vi "ScanParam2DAQParam_old.vi"(11 "AOL_Globals":T1={"Imaging Protocol"=enum."AOL Z-Stack", "Number of POI"=0, "Number of Miniscans"=0, "Number of Trials"=0, "Number of Cycles "=0, "# Averaged Frames"=0, "Laser power (%)"=0, "Pockels (V)"=0.0, "Acquisition Length (sec)"=0.0, "Fill time (us)"=0.0, "POI Dwell time (us)"=0.0, "Miniscan Dwell time per pixel (us)"=0.0, "PMT 1"=0.0, "PMT 2"=0.0, "Back Apperture (mA)"=200.0, "Frame Size"=0, "Center Frequency"=0.0, "Field of View (norm)"=0.0, "DwellTime (us)"=0.0, "Wavelength (nm)"=0.0, "Zoom"=0.0, "AOL Z"=0.0, "AOL Mode"=enum."Raster", "GridXY"=0.0, "GridZ"=0.0, "TriggerPeriod (sec)"=0.0, "Number of Pixels in Miniscan"=0, "Experiment folder path"=path "", "X centre"=0.0, "Y centre"=0.0, "Angle (degrees)"=0.0, "Plane Mode"=0, "Threshold"=[], "Regenerate Chirps"=FALSE, "Rectangle ROI length (pixels)"=0, "Rectangle ROI height (pixels)"=0, "AOD fill"=4900, "StartupDelay"=0, "Samples Wait after Trigger"=5080, "Slip Cycle"=600000, "Add Cycle"=TRUE, "Functional Mode"=enum."Point", "Z Start"=0.0, "Z Stop"=0.0, "# Planes"=0, "Total Pixels"=0, "Variable Miniscan Pixels"=[], "Use Variable Length"=FALSE, "Use Variable Resolution"=FALSE, "Laser power (%) at Z Start"=0, "Laser power (%) at Z Stop"=0, "Ref Z Step"=0, "Ref Dwell Time (us)"=0.0, "Field of View (um)"=175.0} {"Plane Mode" items=["XY Plane", "XZ Plane", "YZ Plane", "arbitraryplane"]; "Frame Size" items=["100X100"=100, "128X128"=128, "200X200"=200, "256X256"=256, "512X512"=512, "1024x1024"=1024, "2048x2048"=2048]; "Back Apperture (mA)" format="%#.6g"; "Pockels (V)" format="%#.6g"; "PMT 2" format="%#.6g"; "PMT 1" format="%#.6g"; "Angle (degrees)" format="%#.6g"; "POI Dwell time (us)" format="%#.6g"}) -> (3 "DAQ Input Parameters(FlexRIO)":T7 {"diff_threshZ" format="%#_11g"; "proportioanl_scale Z" format="%#_15g"; "var_x" format="%#_14g"; "var_y" format="%#_14g"; "scale" format="%#_15g"; "diff_thresh" format="%#_11g"; "proportioanl_scale" format="%#_15g"})   [LabVIEW 2020]
uses:
  AOLdrivers/Controls/UI Imaging Parameters.ctl
  Typedefs/Controls/DAQ Input Parameters(FlexRIO).ctl
  FPGA DAQ/FPGA Typedefs/scan_typr.ctl
  Movement Correction/Typedefs/Control algorithm.ctl
  Typedefs/Controls/AOL_Globals.ctl
  Typedefs/Imaging Protocols enum.ctl
  Typedefs/Frame Size.ctl
  Typedefs/AOL modes.ctl
  Typedefs/Plane Mode.ctl
  Typedefs/Functional Mode.ctl
panel:
  in  "Samples Wait after Trigger(240 MHz)":u16=5500
  in  "AOD fill(240 MHz)":u16=4900
  in  "UI Imaging Parameters":T10={"Frame Size"=200, "Dwell Time (ms)"=0.0, "Wavelength (nm)"=0.0, "Zoom"=0.0, "AOL Mode"=enum."Raster Scanning", "Field of View"=4.35, "Imaging Mode"=enum."Live Imaging", "AOL Z"=0.0, "Averages"=0.0} {"Field of View" items=["FOV1"=4.35, "FOV 2"=5.8, "FOV 3"=8.7]; "Frame Size" items=["20X20"=0, "100X100"=100, "128X128"=128, "200X200"=200, "256X256"=256, "512X512"=512]}
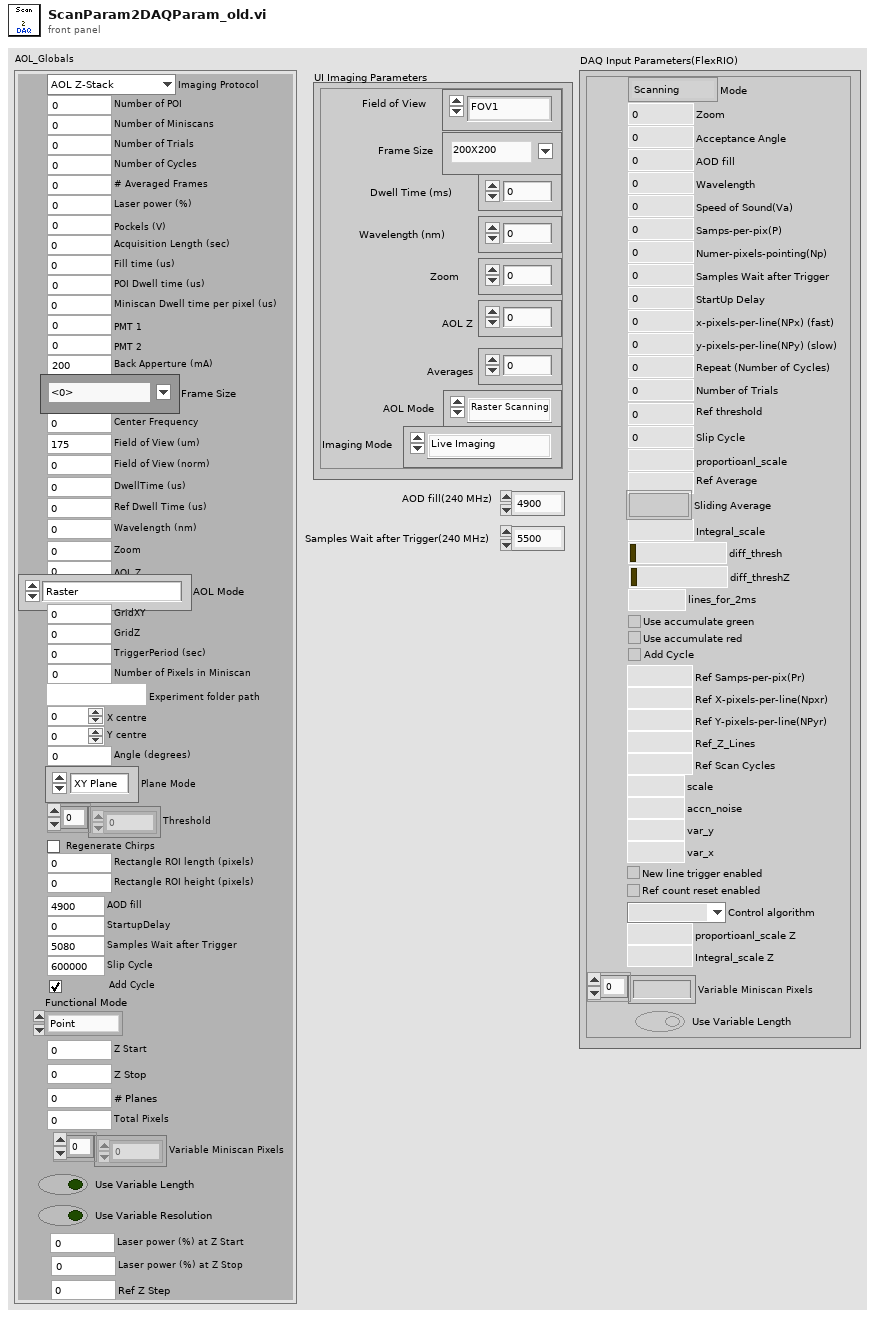
[diagram p1: front panel]
types:
  T1 = typedef "AOL_Globals.ctl" = cluster{"Imaging Protocol":T2, "Number of POI":u16, "Number of Miniscans":u16, "Number of Trials":u16, "Number of Cycles ":u64, "# Averaged Frames":u16, "Laser power (%)":u8, "Pockels (V)":dbl, "Acquisition Length (sec)":dbl, "Fill time (us)":dbl, "POI Dwell time (us)":dbl, "Miniscan Dwell time per pixel (us)":dbl, "PMT 1":dbl, "PMT 2":dbl, "Back Apperture (mA)":dbl, "Frame Size":T3, "Center Frequency":dbl, "Field of View (norm)":dbl, "DwellTime (us)":dbl, "Wavelength (nm)":dbl, "Zoom":dbl, "AOL Z":dbl, "AOL Mode":T4, "GridXY":dbl, "GridZ":dbl, "TriggerPeriod (sec)":dbl, "Number of Pixels in Miniscan":u16, "Experiment folder path":path, "X centre":dbl, "Y centre":dbl, "Angle (degrees)":dbl, "Plane Mode":T5, "Threshold":u16[], "Regenerate Chirps":bool, "Rectangle ROI length (pixels)":u16, "Rectangle ROI height (pixels)":u16, "AOD fill":u16, "StartupDelay":i32, "Samples Wait after Trigger":u16, "Slip Cycle":u32, "Add Cycle":bool, "Functional Mode":T6, "Z Start":dbl, "Z Stop":dbl, "# Planes":i32, "Total Pixels":i32, "Variable Miniscan Pixels":u16[], "Use Variable Length":bool, "Use Variable Resolution":bool, "Laser power (%) at Z Start":u8, "Laser power (%) at Z Stop":u8, "Ref Z Step":i8, "Ref Dwell Time (us)":dbl, "Field of View (um)":dbl}
  T2 = typedef "Imaging Protocols enum.ctl" = enum16{"AOL Z-Stack", "Motor Z Stack", "Functional Acquisition", "Single Plane Acquisition", "Volume Acquisition", "Live Imaging", "Live Plane Imaging", "Live Volume Imaging"}
  T3 = typedef "Frame Size.ctl" = u16
  T4 = typedef "AOL modes.ctl" = enum16{"Raster", "Structural", "Pointing", "Mini Scan", "Alignment"}
  T5 = typedef "Plane Mode.ctl" = u16
  T6 = typedef "Functional Mode.ctl" = enum16{"Point", "Line", "Patch", "Plane", "Volume"}
  T7 = typedef "DAQ Input Parameters(FlexRIO).ctl" = cluster{"Mode":T8, "Zoom":i8, "Acceptance Angle":i8, "AOD fill":u16, "Wavelength":i16, "Speed of Sound(Va)":i8, "Samps-per-pix(P)":i16, "Numer-pixels-pointing(Np)":u32, "Samples Wait after Trigger":u16, "StartUp Delay":i32, "x-pixels-per-line(NPx) (fast)":u16, "y-pixels-per-line(NPy) (slow)":u16, "Repeat (Number of Cycles)":u32, "Number of Trials":u16, "Ref threshold":u16, "Slip Cycle":u32, "proportioanl_scale":fxp<+,16,2>, "Ref Average":u16, "Sliding Average":bool, "Integral_scale":fxp<+/-,16,12>, "diff_thresh":fxp<+/-,16,8>, "diff_threshZ":fxp<+/-,16,8>, "lines_for_2ms":i16, "Use accumulate green":bool, "Use accumulate red":bool, "Add Cycle":bool, "Ref Samps-per-pix(Pr)":i16, "Ref X-pixels-per-line(Npxr)":i16, "Ref Y-pixels-per-line(NPyr)":i16, "Ref_Z_Lines":i16, "Ref Scan Cycles":i32, "scale":fxp<+,16,2>, "accn_noise":fxp<+,16,16>, "var_y":fxp<+,16,4>, "var_x":fxp<+,16,4>, "New line trigger enabled":bool, "Ref count reset enabled":bool, "Control algorithm":T9, "proportioanl_scale Z":fxp<+,16,2>, "Integral_scale Z":fxp<+/-,16,12>, "Variable Miniscan Pixels":u16[], "Use Variable Length":bool}
  T8 = typedef "scan_typr.ctl" = enum16{"Scanning", "Pointing", "Pointing & MC", "Scanning & MC"}
  T9 = typedef "Control algorithm.ctl" = enum16{"PID", "Kalman"}
  T10 = typedef "UI Imaging Parameters.ctl" = cluster{"Frame Size":u16, "Dwell Time (ms)":dbl, "Wavelength (nm)":dbl, "Zoom":dbl, "AOL Mode":enum16{"Raster Scanning", "Structural Imaging", "Functional Imaging", "Alignment Mode", "Mini Scan"}, "Field of View":sgl, "Imaging Mode":enum16{"Live Imaging", "AOL Zstack", "Motor Zstack", "Functional Imaging"}, "AOL Z":sgl, "Averages":dbl}
  T11 = enum16{"Raster Scanning", "Structural Imaging", "Functional Imaging", "Alignment Mode", "Mini Scan"}
  T12 = enum16{"Scanning", "Pointing", "Pointing & MC", "Scanning & MC"}
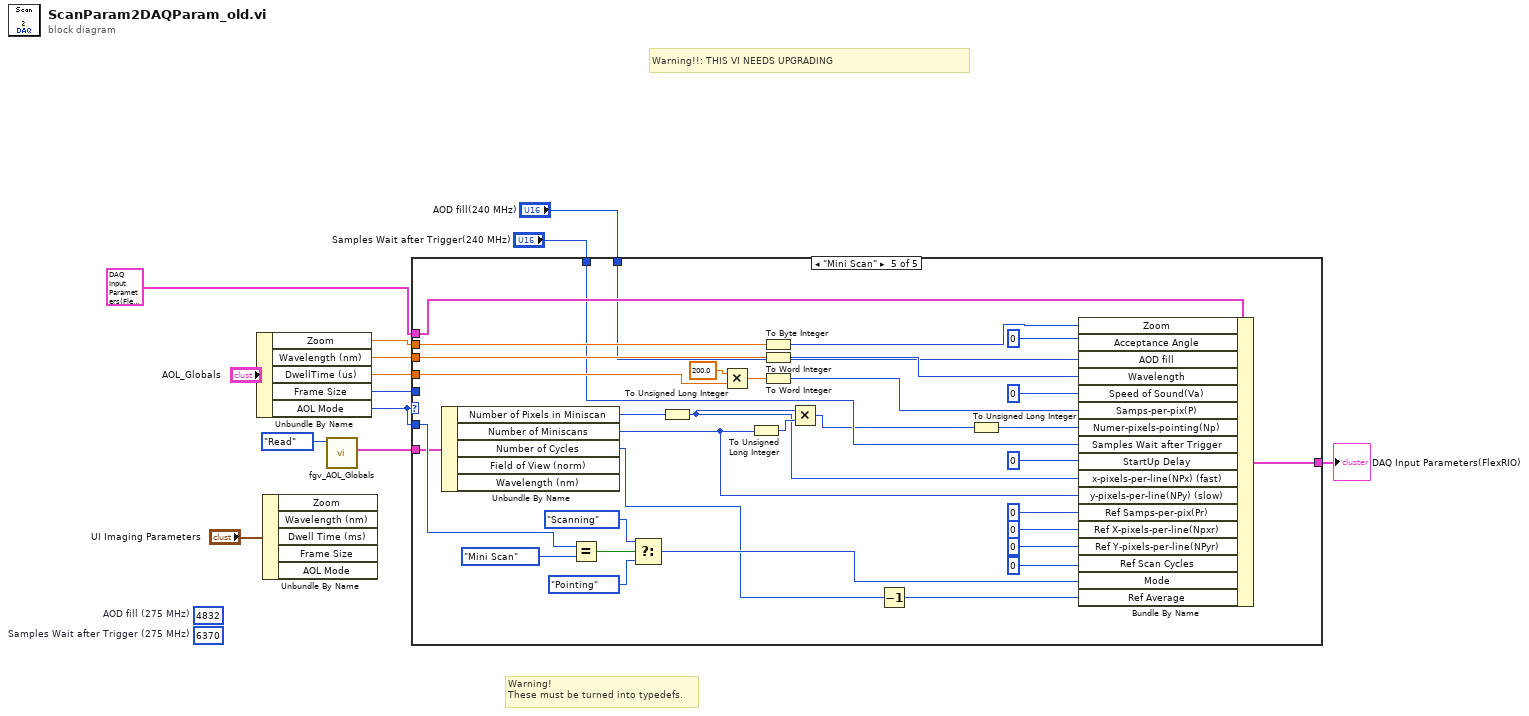
[diagram p0: block diagram]
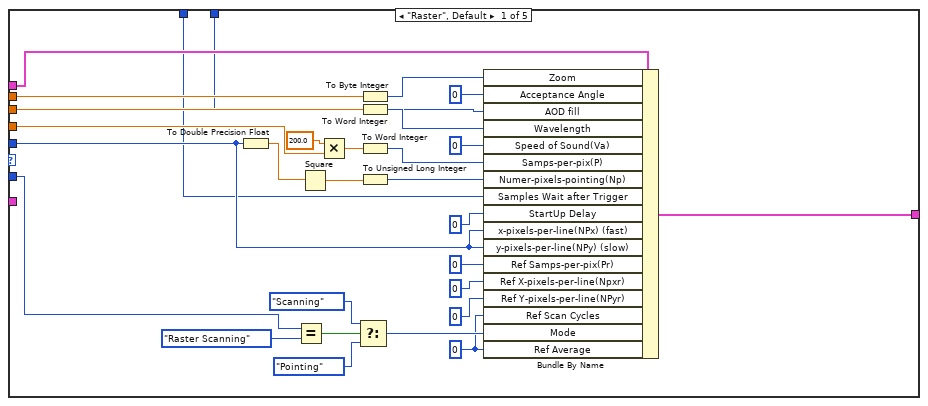
[diagram p2: hidden frame]
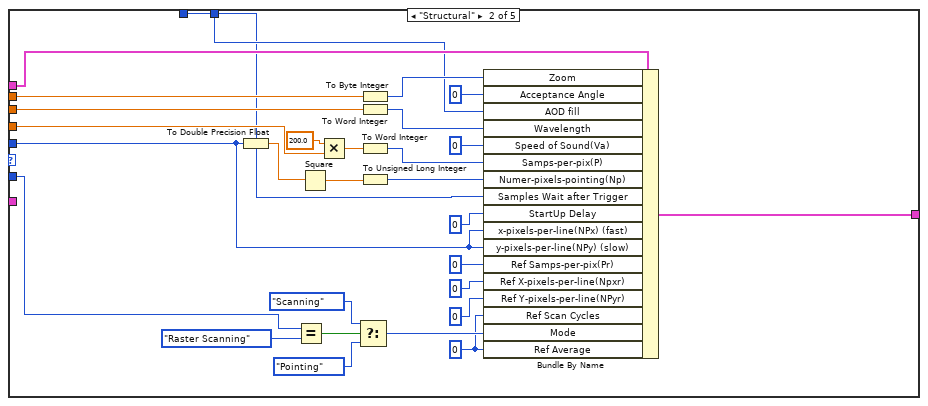
[diagram p3: hidden frame]
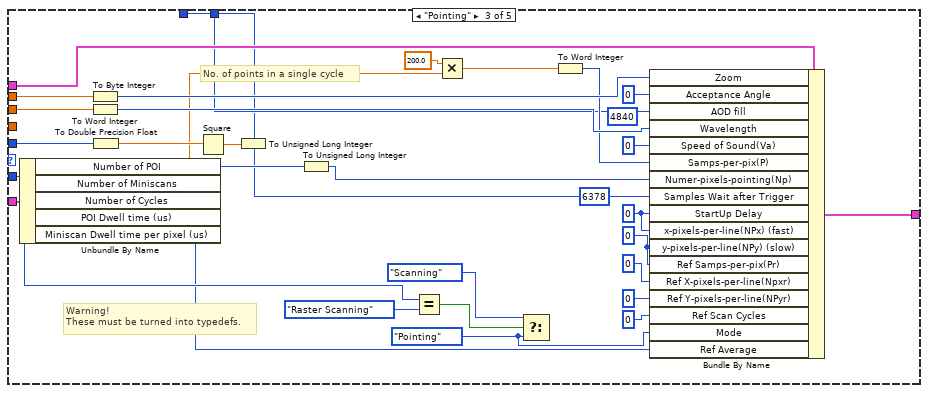
[diagram p4: hidden frame]
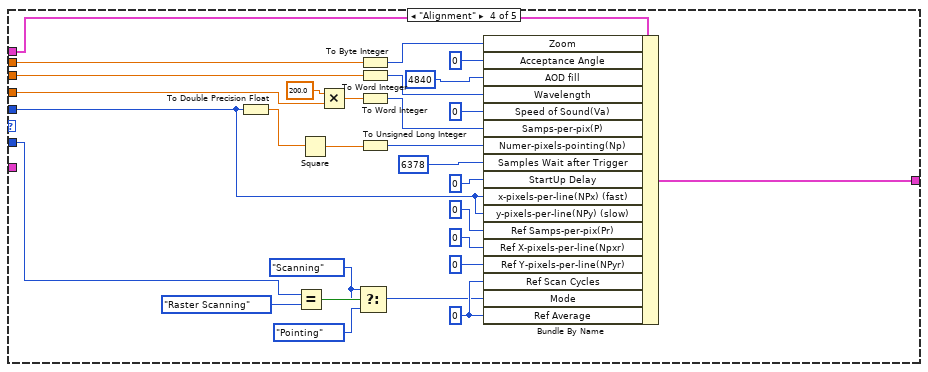
[diagram p5: hidden frame]
diagram:
  (unwired) u16 6370  # Samples Wait after Trigger (275 MHz)
  (unwired) u16 4832  # AOD fill (275 MHz)
  # "Warning!!: THIS VI NEEDS UPGRADING"
  # "Warning!\nThese must be turned into typedefs."
  n1 = Unbundle By Name("AOL_Globals") -> ("Zoom"=w8:dbl, "Wavelength (nm)"=w7:dbl, "DwellTime (us)"=w6:dbl, "Frame Size"=w5:T3, "AOL Mode"=w4:T4)
  n2 = Unbundle By Name("UI Imaging Parameters") -> ()  [unwired: 5 out]
  n3 = call "fgv_AOL_Globals.vi"("Function"=enum16{"Intialize", "Write", "Read", "Clear"}."Read") -> ("AOL_Globals"=w3:T1)  [unwired: 9 in, 1 out]
  n4 = case shown="\"Mini Scan\"" w4 {
    tunnel: T7 data[162B] ("DAQ Input Parameters(FlexRIO)") -> [w42 w71 w102 w106 w164]
    tunnel: w4 -> [w31 w60 w94 w121 w154]
    tunnel: [w29 w58 w92 w119 w152] -> w11
    tunnel: w8 -> [w22 w51 w86 w112 w149]
    tunnel: w6 -> [w20 w49 _ w110 w148]
    tunnel: w7 -> [w19 w48 w84 w109 w147]
    tunnel: w5 -> [w18 w47 w83 w108 _]
    tunnel: w3 -> [_ _ w80 _ w144]
    tunnel: "AOD fill(240 MHz)" -> [w15 w44 w73 _ w141]
    tunnel: "Samples Wait after Trigger(240 MHz)" -> [w14 w43 w72 _ w140]
    frame "Raster", Default {
      w16 = 0 ("Ref Scan Cycles")
      n5 = To Double Precision Float(number=w18) -> (double precision float=w24:dbl)
      n6 = Equal?(x=w31, y=T11."Raster Scanning" ("AOL Mode")) -> (x = y?=w30:bool)
      n7 = Square(x=w24) -> (x^2=w28:dbl)
      n8 = Multiply(x=200.0, y=w20) -> (x*y=w27:dbl)
      n9 = Select(t=T12."Scanning" ("Mode"), s=w30, f=T12."Pointing" ("Mode")) -> (s? t:f=w17:T12)
      n10 = To Byte Integer(number=w22) -> (8bit integer=w41:i8)
      n11 = To Word Integer(number=w19) -> (16bit integer=w40:i16)
      n12 = To Word Integer(number=w27) -> (16bit integer=w25:i16)
      n13 = To Unsigned Long Integer(number=w28) -> (unsigned 32bit integer=w23:u32)
      n14 = Bundle By Name(cluster=w42, "Zoom"=w41, "Acceptance Angle"=i8 0, "AOD fill"=w15, "Wavelength"=w40, "Speed of Sound(Va)"=i8 0, "Samps-per-pix(P)"=w25, "Numer-pixels-pointing(Np)"=w23, "Samples Wait after Trigger"=w14, "StartUp Delay"=0, "x-pixels-per-line(NPx) (fast)"=w18, "y-pixels-per-line(NPy) (slow)"=w18, "Ref Samps-per-pix(Pr)"=i16 0, "Ref X-pixels-per-line(Npxr)"=i16 0, "Ref Y-pixels-per-line(NPyr)"=i16 0, "Ref Scan Cycles"=w16, "Mode"=w17, "Ref Average"=w16) -> (w29:T7)
    }
    frame "Structural" {
      w45 = 0 ("Ref Scan Cycles")
      n15 = To Double Precision Float(number=w47) -> (double precision float=w53:dbl)
      n16 = Equal?(x=w60, y=T11."Raster Scanning" ("AOL Mode")) -> (x = y?=w59:bool)
      n17 = Square(x=w53) -> (x^2=w57:dbl)
      n18 = Multiply(x=200.0, y=w49) -> (x*y=w56:dbl)
      n19 = Select(t=T12."Scanning" ("Mode"), s=w59, f=T12."Pointing" ("Mode")) -> (s? t:f=w46:T12)
      n20 = To Byte Integer(number=w51) -> (8bit integer=w70:i8)
      n21 = To Word Integer(number=w48) -> (16bit integer=w69:i16)
      n22 = To Word Integer(number=w56) -> (16bit integer=w54:i16)
      n23 = To Unsigned Long Integer(number=w57) -> (unsigned 32bit integer=w52:u32)
      n24 = Bundle By Name(cluster=w71, "Zoom"=w70, "Acceptance Angle"=i8 0, "AOD fill"=w44, "Wavelength"=w69, "Speed of Sound(Va)"=i8 0, "Samps-per-pix(P)"=w54, "Numer-pixels-pointing(Np)"=w52, "Samples Wait after Trigger"=w43, "StartUp Delay"=0, "x-pixels-per-line(NPx) (fast)"=w47, "y-pixels-per-line(NPy) (slow)"=w47, "Ref Samps-per-pix(Pr)"=i16 0, "Ref X-pixels-per-line(Npxr)"=i16 0, "Ref Y-pixels-per-line(NPyr)"=i16 0, "Ref Scan Cycles"=w45, "Mode"=w46, "Ref Average"=w45) -> (w58:T7)
    }
    frame "Pointing" {
      (unwired) u16 6378 ("Samples Wait after Trigger(240 MHz)")
      (unwired) u16 4840 ("AOD fill(240 MHz)")
      w74 = T12."Pointing" ("Mode")
      w81 = i16 0 ("Ref Samps-per-pix(Pr)")
      w82 = 0 ("StartUp Delay")
      # "Warning!\nThese must be turned into typedefs."
      # "No. of points in a single cycle"
      n25 = Unbundle By Name(w80) -> ("Number of POI"=w79:u16, "Number of Cycles"=w77:u64, "POI Dwell time (us)"=w75:dbl)  [unwired: 2 out]
      n26 = To Byte Integer(number=w86) -> (8bit integer=w101:i8)
      n27 = To Word Integer(number=w84) -> (16bit integer=w100:i16)
      n28 = To Double Precision Float(number=w83) -> (double precision float=w87:dbl)
      n29 = Square(x=w87) -> (x^2=w91:dbl)
      n30 = To Unsigned Long Integer(number=w91) -> ()  [unwired: 1 out]
      n31 = To Unsigned Long Integer(number=w79) -> (unsigned 32bit integer=w78:u32)
      n32 = Equal?(x=w94, y=T11."Raster Scanning" ("AOL Mode")) -> (x = y?=w93:bool)
      n33 = Multiply(x=200.0, y=w75) -> (x*y=w90:dbl)
      n34 = Select(t=T12."Scanning" ("Mode"), s=w93, f=w74) -> ()  [unwired: 1 out]
      n35 = To Word Integer(number=w90) -> (16bit integer=w88:i16)
      n36 = Bundle By Name(cluster=w102, "Zoom"=w101, "Acceptance Angle"=i8 0, "AOD fill"=w73, "Wavelength"=w100, "Speed of Sound(Va)"=i8 0, "Samps-per-pix(P)"=w88, "Numer-pixels-pointing(Np)"=w78, "Samples Wait after Trigger"=w72, "StartUp Delay"=w82, "x-pixels-per-line(NPx) (fast)"=w82, "y-pixels-per-line(NPy) (slow)"=w81, "Ref Samps-per-pix(Pr)"=w81, "Ref X-pixels-per-line(Npxr)"=i16 0, "Ref Y-pixels-per-line(NPyr)"=i16 0, "Ref Scan Cycles"=0, "Mode"=w74, "Ref Average"=w77) -> (w92:T7)
    }
    frame "Alignment" {
      w105 = T12."Scanning" ("Mode")
      w107 = 0 ("Ref Scan Cycles")
      n37 = To Double Precision Float(number=w108) -> (double precision float=w114:dbl)
      n38 = Equal?(x=w121, y=T11."Raster Scanning" ("AOL Mode")) -> (x = y?=w120:bool)
      n39 = Square(x=w114) -> (x^2=w118:dbl)
      n40 = Multiply(x=200.0, y=w110) -> (x*y=w117:dbl)
      n41 = Select(t=w105, s=w120, f=T12."Pointing" ("Mode")) -> ()  [unwired: 1 out]
      n42 = To Byte Integer(number=w112) -> (8bit integer=w130:i8)
      n43 = To Word Integer(number=w109) -> (16bit integer=w129:i16)
      n44 = To Word Integer(number=w117) -> (16bit integer=w115:i16)
      n45 = To Unsigned Long Integer(number=w118) -> (unsigned 32bit integer=w113:u32)
      n46 = Bundle By Name(cluster=w106, "Zoom"=w130, "Acceptance Angle"=i8 0, "AOD fill"=u16 4840 ("AOD fill(240 MHz)"), "Wavelength"=w129, "Speed of Sound(Va)"=i8 0, "Samps-per-pix(P)"=w115, "Numer-pixels-pointing(Np)"=w113, "Samples Wait after Trigger"=u16 6378 ("Samples Wait after Trigger(240 MHz)"), "StartUp Delay"=0, "x-pixels-per-line(NPx) (fast)"=w108, "y-pixels-per-line(NPy) (slow)"=w108, "Ref Samps-per-pix(Pr)"=i16 0, "Ref X-pixels-per-line(Npxr)"=i16 0, "Ref Y-pixels-per-line(NPyr)"=i16 0, "Ref Scan Cycles"=w107, "Mode"=w105, "Ref Average"=w107) -> (w119:T7)
    }
    frame "Mini Scan" {
      n47 = Unbundle By Name(w144) -> ("Number of Pixels in Miniscan"=w138:u16, "Number of Miniscans"=w137:u16, "Number of Cycles"=w143:u64)  [unwired: 2 out]
      n48 = Equal?(x=w154, y=AOL_modes."Mini Scan" ("AOL Mode")) -> (x = y?=w153:bool)
      n49 = Select(t=T12."Scanning" ("Mode"), s=w153, f=T12."Pointing" ("Mode")) -> (s? t:f=w146:T12)
      n50 = To Unsigned Long Integer(number=w138) -> (unsigned 32bit integer=w134:u32)
      n51 = Multiply(x=200.0, y=w148) -> (x*y=w151:dbl)
      n52 = To Unsigned Long Integer(number=w137) -> (unsigned 32bit integer=w135:u32)
      n53 = To Byte Integer(number=w149) -> (8bit integer=w142:i8)
      n54 = To Word Integer(number=w147) -> (16bit integer=w163:i16)
      n55 = To Word Integer(number=w151) -> (16bit integer=w132:i16)
      n56 = Multiply(x=w134, y=w135) -> (x*y=w136:u32)
      n57 = Decrement(x=w143) -> (x-1=w131:u64)
      n58 = To Unsigned Long Integer(number=w136) -> (unsigned 32bit integer=w139:u32)
      n59 = Bundle By Name(cluster=w164, "Zoom"=w142, "Acceptance Angle"=i8 0, "AOD fill"=w141, "Wavelength"=w163, "Speed of Sound(Va)"=i8 0, "Samps-per-pix(P)"=w132, "Numer-pixels-pointing(Np)"=w139, "Samples Wait after Trigger"=w140, "StartUp Delay"=0, "x-pixels-per-line(NPx) (fast)"=w134, "y-pixels-per-line(NPy) (slow)"=w137, "Ref Samps-per-pix(Pr)"=i16 0, "Ref X-pixels-per-line(Npxr)"=i16 0, "Ref Y-pixels-per-line(NPyr)"=i16 0, "Ref Scan Cycles"=0, "Mode"=w146, "Ref Average"=w131) -> (w152:T7)
    }
  }
  "DAQ Input Parameters(FlexRIO)" <- w11
